vi "servo define.vi"() -> ()   [LabVIEW 2013]
panel:
  in  "invalid PWD":i32=-1
  in  "ARM_MAX":i32=180
  in  "ARM_MID":i32=90
  in  "ARM_MIN":i32
  in  "BASE_STOP":i32=1475
  in  "Arm ID":i32=7
  in  "Base ID":i32=6
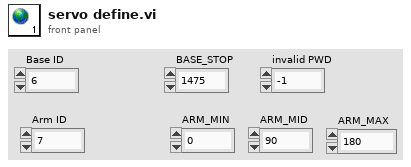
[diagram p1: front panel]
diagram:
